vi "Performance Values.vi"(8 "error in (no error)":errorcluster, 11 "Linux System SAL in":refnum<class "Linux System SAL.lvclass">) -> (0 "error out":errorcluster, 2 "Performance Values":T1)   [LabVIEW 2020, in "Volatus.lvlib" / "Linux System SAL.lvclass"]
uses:
  Linux System SAL.lvclass
  Linux System SAL.lvclass/Linux System SAL.ctl
  System SAL/Performance Values.ctl
  System SAL/System SAL.lvclass
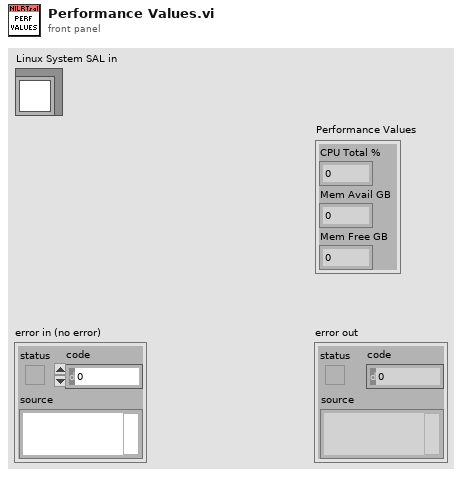
[diagram p1: front panel]
types:
  T1 = typedef "Volatus.lvlib/System SAL.lvclass/Performance Values.ctl" = cluster{"CPU Total %":dbl, "Mem Avail GB":dbl, "Mem Free GB":dbl}
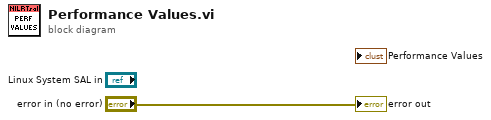
[diagram p0: block diagram]
diagram:
  "error out" <- "error in (no error)"
